vi "Robot Main.vi"() -> ()   [LabVIEW 2017]
doc: "Robot Main serves as the primary scheduler for your command and control robotics program. It should not be necessary to modify this VI. Instead, you should add your code to the VIs called from Robot Main - Teleop, Autonomous, and SubSystems."
uses:
  <vilib>/Rock Robotics/WPI/Camera/WPI_CameraImageSize.ctl
  <vilib>/Rock Robotics/SystemInterfaces/NetworkCommunication/NetComm_UsageReport_ResourceType.ctl
  <vilib>/Rock Robotics/WPI/ThirdParty/Sensors/navX/_Processing Loop/FRIC_navX_Internal_SPI_ProcessingLoop.vi
  Framework/Robot Global Data.vi
panel:
  in  "Image Size":T1=enum."320x240"
  in  "Enable Vision":bool
  in  "Finish":bool
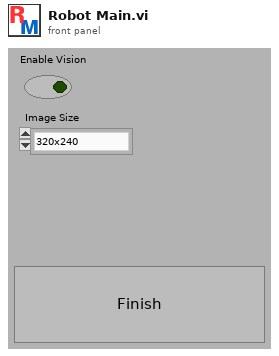
[diagram p1: front panel]
types:
  T1 = typedef "WPI_CameraImageSize.ctl" = enum16{"640x480", "320x240", "160x120", "Custom"}
  T2 = typedef "NetComm_UsageReport_ResourceType.ctl" = enum8{"Controller", "Module", "Language", "CANPlugin", "Accelerometer", "ADXL345", "AnalogChannel", "AnalogTrigger", "AnalogTriggerOutput", "CANJaguar", "Compressor", "Counter", "Dashboard", "DigitalInput", "DigitalOutput", "DriverStationCIO", "DriverStationEIO", "DriverStationLCD", "Encoder", "GearTooth", "Gyro", "I2C", "Framework", "Jaguar", "Joystick", "Kinect", "KinectStick", "PIDController", "Preferences", "PWM", "Relay", "RobotDrive", "SerialPort", "Servo", "Solenoid", "SPI", "Task", "Ultrasonic", "Victor", "Button", "Command", "AxisCamera", "PCVideoServer", "SmartDashboard", "Talon", "HiTechnicColorSensor", "HiTechnicAccel", "HiTechnicCompass", "SRF08", "AnalogOutput", "Victor SP", "Talon SRX", "CAN Talon SRX", "ADXL362 Accel", "ADXRS450 Gyro", "Rev SPARK", "Mindsensors SD540", "Digital Filter", "ADIS16448", "PDP", "PCM", "PigeonIMU", "Nidec Brushless", "CTRE CANifier", "CTRE Future 0", "CTRE Future 1", "CTRE Future 2", "CTRE Future 3", "CTRE Future 4", "CTRE Future 5", "CTRE Future 6"}
  T3 = typedef "WPI_DriverStationMatch Info.ctl" = cluster{"Autonomous Elapsed Seconds":dbl, "TeleOp Elapsed Seconds":dbl, "Disabled Elapsed Seconds":dbl, "Visited Autonomous":bool, "Visited TeleOp":bool, "Visited Disabled":bool, "Autonomous Settings":cluster{"Autonomous Style":enum16{"Iterative", "Independent"}, "VI Refnum":refnum<vi>}}
  T4 = typedef "WPI_DriverStationDerivedRobotMode.ctl" = enum16{"Init", "Execute", "Stop"}
  T5 = typedef "WPI_DriverStationRobotMode2.ctl" = enum16{"Autonomous Disabled", "Autonomous Enabled", "Teleop Disabled", "Teleop Enabled", "Disconnected", "Finish", "Test Disabled", "Test Enabled", "Emergency Stopped"}
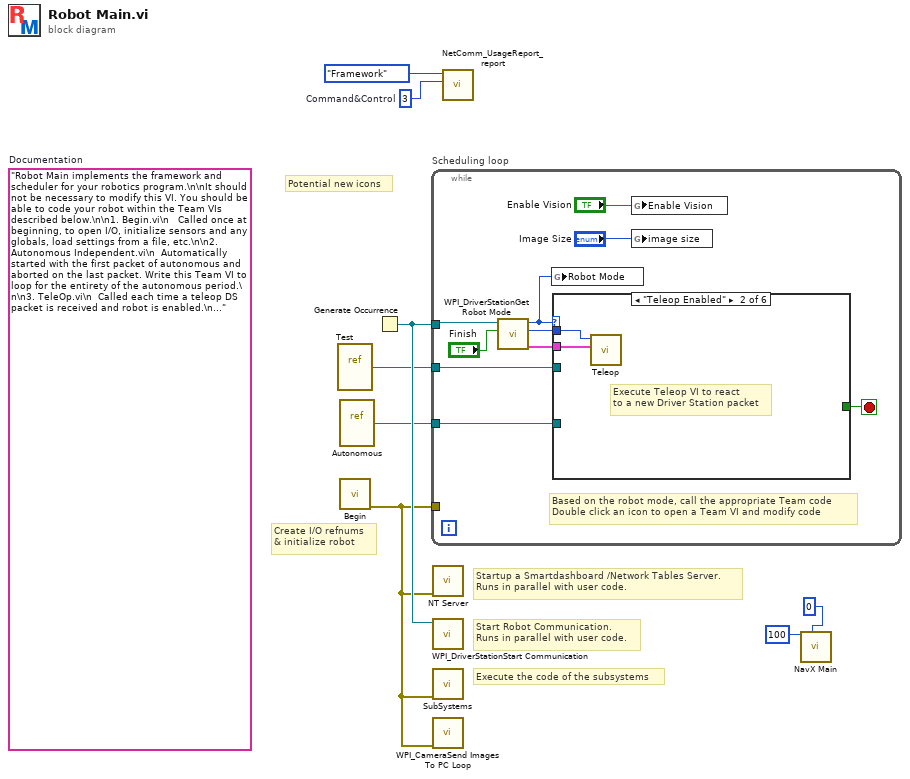
[diagram p0: block diagram]
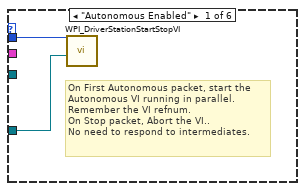
[diagram p2: hidden frame]
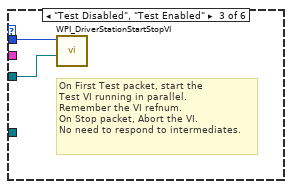
[diagram p3: hidden frame]
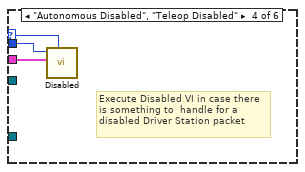
[diagram p4: hidden frame]
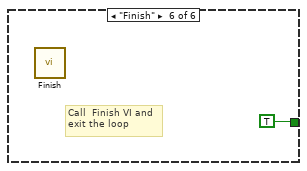
[diagram p6: hidden frame]
diagram:
  w4 = u8 3  # Command&Control
  (unwired) "Robot Main implements the framework and scheduler for your robotics program.\n\nIt should not be necessary to modify this VI. You should be able to code your robot within the Team VIs described below.\n\n1. Begin.vi\n   Called once at beginning, to open I/O, initialize sensors and any globals, load settings from a file, etc.\n\n2. Autonomous Independent.vi\n  Automatically started with the first packet of autonomous and aborted on the last packet. Write this Team VI to loop for the entirety of the autonomous period.\n\n3. TeleOp.vi\n  Called each time a teleop DS packet is received and robot is enabled.\n\n4. Disabled.vi\n  Called each time a packet is received and the robot is disabled.\n\n5. Test.vi\n  Called Automatically started with the first test packet and aborted on the last. Modify this VI to carry out robot and sensor validation tests.\n\n6. Vision.vi\n  A parallel loop that acquires and processes camera images.\n\n7. PeriodicTasks.vi\n  Parallel loops running at user-defined rates.\n\n8. Finish.vi\n  Called before exiting, so you can save data, clean up I/O, etc.\n"  # Documentation
  # "Potential new icons"
  # "Startup a Smartdashboard /Network Tables Server.\nRuns in parallel with user code."
  # "Execute the code of the subsystems"
  # "Create I/O refnums\n& initialize robot"
  # "Start Robot Communication.\nRuns in parallel with user code."
  n1 = vi-ref "Test.vi"() -> (w6:refnum<vi>)
  n2 = vi-ref "Autonomous.vi"() -> (w7:refnum<vi>)
  n3 = call "Begin.vi"() -> ("error out"=w3:errorcluster)  [unwired: 2 in, 9 out]
  n4 = Generate Occurrence() -> (w8:refnum<k4>)
  n5 = while "Scheduling loop" {
    tunnel: w8 -> [w17]
    tunnel: w3 -> [_]
    tunnel: w7 -> [w12]
    tunnel: w6 -> [w10]
    stop <- w14 stop-if-true
    # "Based on the robot mode, call the appropriate Team code\nDouble click an icon to open a Team VI and modify code"
    n6 = call <vilib>:"WPI_DriverStationGet Robot Mode.vi"("Finish"="Finish", "DS Occurrence"=w17) -> ("Match Info out"=w15:T3, "Call Context"=w18:T4, "Robot Mode"=w9:T5)  [unwired: 7 out]
    n7 = global write "Robot Global Data.vi" "Robot Mode"(w9) -> ()
    n8 = case shown="\"Teleop Enabled\"" w9 {
      selector: w9 -> [_ _ _ w25 _ _]
      tunnel: w18 -> [w20 w22 w24 w27 _ _]
      tunnel: w15 -> [_ w21 _ w26 _ _]
      tunnel: [_ _ _ _ _ TRUE] -> w14
      tunnel: w12 -> [w19 _ _ _ _ _]
      tunnel: w10 -> [_ _ w23 _ _ _]
      frame "Autonomous Enabled" {
        # "On First Autonomous packet, start the\nAutonomous VI running in parallel.\nRemember the VI refnum.\nOn Stop packet, Abort the VI..\nNo need to respond to intermediates."
        n9 = call <vilib>:"WPI_DriverStationStartStopVI.vi"("VI in"=w19, "Call Context"=w20) -> ()  [unwired: 10 in]
      }
      frame "Teleop Enabled" {
        # "Execute Teleop VI to react\nto a new Driver Station packet"
        n10 = call "Teleop.vi"("Match Info"=w21, "Call Context"=w22) -> ()  [unwired: 1 in, 9 out]
      }
      frame "Test Disabled", "Test Enabled" {
        # "On First Test packet, start the\nTest VI running in parallel.\nRemember the VI refnum.\nOn Stop packet, Abort the VI.\nNo need to respond to intermediates."
        n11 = call <vilib>:"WPI_DriverStationStartStopVI.vi"("VI in"=w23, "Call Context"=w24) -> ()  [unwired: 10 in]
      }
      frame "Autonomous Disabled", "Teleop Disabled" {
        # "Execute Disabled VI in case there\nis something to  handle for a\ndisabled Driver Station packet"
        n12 = call "Disabled.vi"("Robot Mode"=w25, "Match Info"=w26, "Call Context"=w27) -> ()  [unwired: 1 in, 8 out]
      }
      frame "Disconnected", Default {
        # "Driver Station packet didn't arrive.\nPossibly useful for diagnostics"
      }
      frame "Finish" {
        # "Call  Finish VI and\nexit the loop"
        n13 = call "Finish.vi"() -> ()  [unwired: 1 in, 7 out]
      }
    }
    n14 = global write "Robot Global Data.vi" "Enable Vision"("Enable Vision") -> ()
    n15 = global write "Robot Global Data.vi" "image size"("Image Size") -> ()
  }
  n16 = call <vilib>:"NT Server.vi"("error in (no error)"=w3) -> ()  [unwired: 11 in]
  n17 = call <vilib>:"WPI_DriverStationStart Communication.vi"("occurrence"=w8) -> ()  [unwired: 1 in, 10 out]
  n18 = call "SubSystems.vi"("error in"=w3) -> ()  [unwired: 11 in]
  n19 = call <vilib>:"WPI_CameraSend Images To PC Loop.vi"("error in (no error)"=w3) -> ()  [unwired: 11 in]
  n20 = call <vilib>:"NetComm_UsageReport_report.vi"("Instance Number"=w4, "Resource Type"=NetComm_UsageReport_ResourceType."Framework") -> ()  [unwired: 10 in]
  n21 = call-poly <vilib>:"NavX Main.vi"("Device Number"=0, "Rate (4Hz-200Hz)"=100) -> ()  [unwired: 10 in]
